vi "Read O3.vi"(8 "error in (no error)":errorcluster, 11 "xData in":refnum<class "xData.lvclass">) -> (0 "error out":errorcluster, 2 "O3":bool, 3 "xData out":refnum<class "xData.lvclass">)   [LabVIEW 2014, in "xData.lvclass"]
uses:
  xData.lvclass
  xData.lvclass/xData.ctl
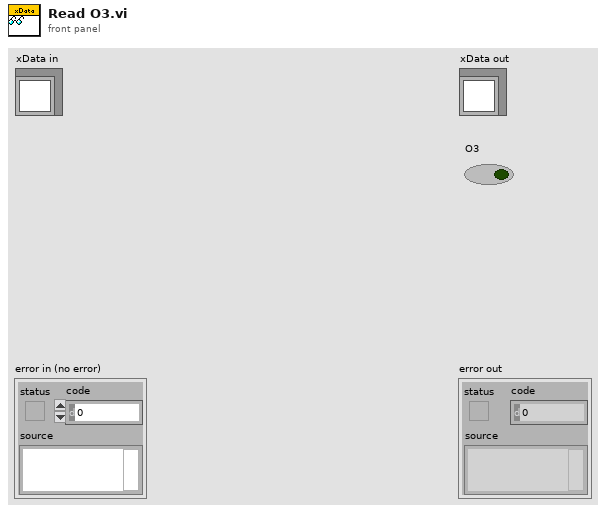
[diagram p1: front panel]
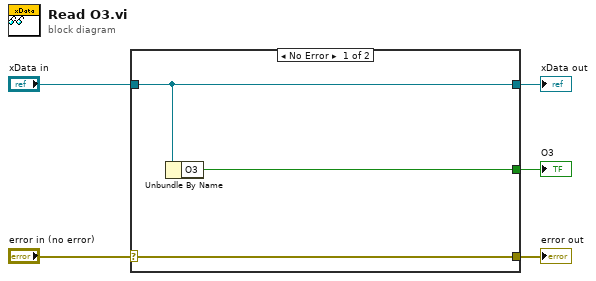
[diagram p0: block diagram]
diagram:
  n1 = case shown="No Error" "error in (no error)" {
    selector: "error in (no error)" -> [w8 w9]
    tunnel: [w8 w9] -> w4
    tunnel: [w7 w10] -> w2
    tunnel: "xData in" -> [w7 w10]
    tunnel: [w6 _] -> w1
    frame No Error {
      n2 = Unbundle By Name(w7) -> ("O3"=w6:bool)
    }
    frame Error {
    }
  }
  "error out" <- w4
  "xData out" <- w2
  "O3" <- w1
